vi "IncrementFrameNumber.vi"(8 "error in (no error)":errorcluster, 11 "reference in":refnum<class "Camera_IMAQdx.lvclass">) -> (0 "error out":errorcluster, 2 "Frame Number":u32, 3 "reference out":refnum<class "Camera_IMAQdx.lvclass">)   [LabVIEW 2017, in "Camera_IMAQdx.lvclass"]
uses:
  Camera_IMAQdx.lvclass
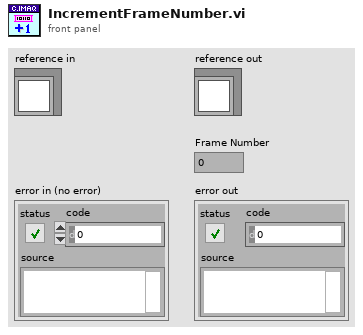
[diagram p1: front panel]
types:
  T1 = typedef "Camera_IMAQdx.lvclass/ObjectAttributes.ctl" = cluster{"Configuration":T2, "Session":T4, "Connected":bool, "Image":T5, "Frame Number":u32}
  T2 = typedef "Camera_IMAQdx.lvclass/Configuration--Cluster.ctl" = cluster{"Camera Interface Name":string, "Number of Buffers":u32, "Image Name":string, "Image Type":T3}
  T3 = typedef "Image Type" = u32
  T4 = typedef "IMAQdx.ctl" = refnum<k21>
  T5 = typedef "IMAQ Image.ctl" = refnum<image>
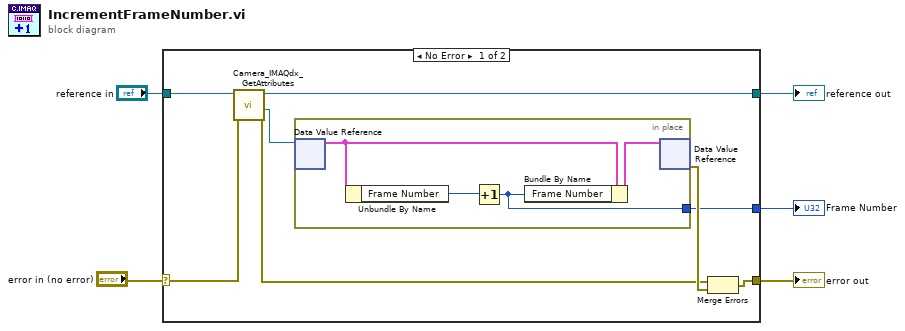
[diagram p0: block diagram]
diagram:
  n1 = case shown="No Error" "error in (no error)" {
    selector: "error in (no error)" -> [w7 w18]
    tunnel: [w12 w18] -> w5
    tunnel: [w10 w19] -> w4
    tunnel: "reference in" -> [w9 w19]
    tunnel: [w6 _] -> w1
    frame No Error {
      n2 = call "Camera_IMAQdx_GetAttributes.vi"("error in (no error)"=w7, "reference in"=w9) -> ("error out"=w11:errorcluster, "DataRef"=w8:refnum<data-value>, "reference out"=w10:refnum<class "Camera_IMAQdx.lvclass">)  [unwired: 6 in, 1 out]
      n3 = in-place {
        in-place-border: [w14] -> w6
        n4 = in-place-dvr #1(w8) -> (w16:T1)  [unwired: 1 out]
        n5 = Unbundle By Name(w16) -> ("Frame Number"=w15:u32)
        n6 = Increment(x=w15) -> (x+1=w14:u32)
        n7 = Bundle By Name(cluster=w16, "Frame Number"=w14) -> (w17:T1)
        n8 = in-place-dvr #1(w17) -> (w13:errorcluster)  [unwired: 1 out]
      }
      n9 = Merge Errors(w11, w13) -> (w12:errorcluster)
    }
    frame Error {
    }
  }
  "error out" <- w5
  "reference out" <- w4
  "Frame Number" <- w1
